vi "Label To Parameters.vi"(8 "error in":errorcluster, 11 "label ref":T4 format="%.0x") -> (0 "error out":errorcluster, 2 "parameters":T1[](array[typedef]), 3 "label ref out":T4 format="%.0x")   [LabVIEW 2020, in "Ballard ARINC 429 Scripting.lvlib"]
uses:
  Ballard ARINC 429 Scripting.lvlib
  Encoding and Decoding/Encoding.ctl
  Encoding and Decoding/Encoding and Decoding.lvlib
  Shared/Parameter Definition.ctl
  Shared/VS Channel Definition for Parameter.ctl
  ARINC 429/ARINC 429 Scripting.lvlib
  <vilib>/NI VeriStand/Custom Device API/Custom Device Item Ref.ctl
  <vilib>/NI VeriStand/Custom Device API/Custom Device API.lvlib
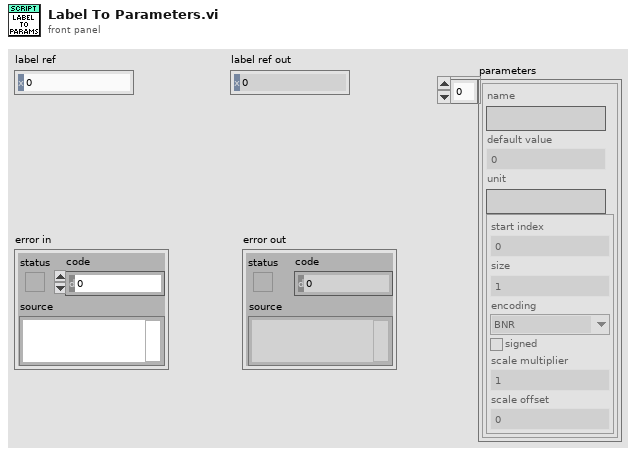
[diagram p1: front panel]
types:
  T1 = typedef "VS Channel Definition for Parameter.ctl" = cluster{"name":string, "default value":dbl, "unit":string, "Parameter":T2}
  T2 = typedef "Parameter Definition.ctl" = cluster{"start index":i32, "size":i32, "encoding":T3, "signed":bool, "scale multiplier":dbl, "scale offset":dbl}
  T3 = typedef "Encoding and Decoding.lvlib/Encoding.ctl" = enum16{"BNR", "BCD", "Discrete"}
  T4 = typedef "Custom Device API.lvlib/Custom Device Item Ref.ctl" = u64
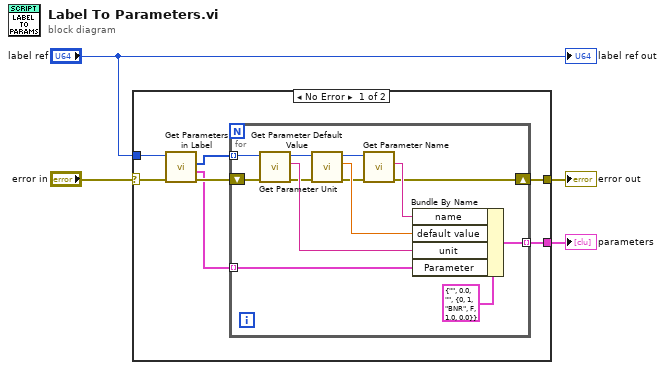
[diagram p0: block diagram]
diagram:
  n1 = case shown="No Error" "error in" {
    selector: "error in" -> [w6 w25]
    tunnel: "label ref" -> [w5 _]
    tunnel: [w8 w25] -> w4
    tunnel: [w7 _] -> w1
    frame No Error {
      n2 = call "Get Parameters in Label.vi"("error in"=w6, "label ref"=w5) -> ("error out"=w11:errorcluster, "parameter definitions"=w10:T2[], "parameter references"=w9:T4[])  [unwired: 6 in, 1 out]
      n3 = for {
        shift-right: [w12] -> w8
        shift-left: w11 -> [w21]
        tunnel: w10 -> [w23] mode=indexing
        tunnel: [w22] -> w7 mode=indexing
        tunnel: w9 -> [w20] mode=indexing
        n4 = call "Get Parameter Unit.vi"("error in"=w21, "parameter ref"=w20) -> ("error out"=w18:errorcluster, "unit"=w19:string, "parameter ref out"=w17:T4)  [unwired: 7 in]
        n5 = call "Get Parameter Default Value.vi"("error in"=w18, "parameter ref"=w17) -> ("error out"=w15:errorcluster, "Default Value (Scaled)"=w16:dbl, "parameter ref out"=w14:T4)  [unwired: 7 in]
        n6 = call "Get Parameter Name.vi"("error in"=w15, "parameter ref"=w14) -> ("error out"=w12:errorcluster, "name"=w13:string)  [unwired: 7 in, 1 out]
        n7 = Bundle By Name(cluster=T1 {"name"="", "default value"=0.0, "unit"="", "Parameter"={"start index"=0, "size"=1, "encoding"=enum."BNR", "signed"=FALSE, "scale multiplier"=1.0, "scale offset"=0.0}} ("channel parameter"), "name"=w13, "default value"=w16, "unit"=w19, "Parameter"=w23) -> (w22:T1)
      }
    }
    frame Error {
    }
  }
  "error out" <- w4
  "parameters" <- w1
  "label ref out" <- "label ref"
